vi "grab_video_in_parallel.vi"() -> ()   [LabVIEW 2015]
uses:
  video_global.vi
  <vilib>/LVH/AR Drone Toolkit/AR Drone.lvlib
panel:
  in  "stop 2":bool
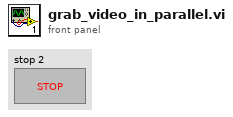
[diagram p1: front panel]
types:
  T1 = typedef "AR Drone.lvlib/AR Drone Resource.ctl" = cluster{"UDP Control Connection":refnum<k16>, "UDP NavData Connection":refnum<k16>, "UDP Video Connection (Drone 1.0)":refnum<k16>, "TCP Video Connection (Drone 2.0)":refnum<k5>, "TCP Control Port Connection":refnum<k5>, "Drone IP address":string, "Drone Command Port":u16, "Drone NavData Port":u16, "Drone Vid Stream Port":u16, "Drone TCP Control Port":u16, "Home IP address":string, "Home Command Port":u16, "Home NavData Port":u16, "Home Vid Stream Port":u16, "Drone Version":i32, "Drone Index":i32, "Command Sequence":i32}
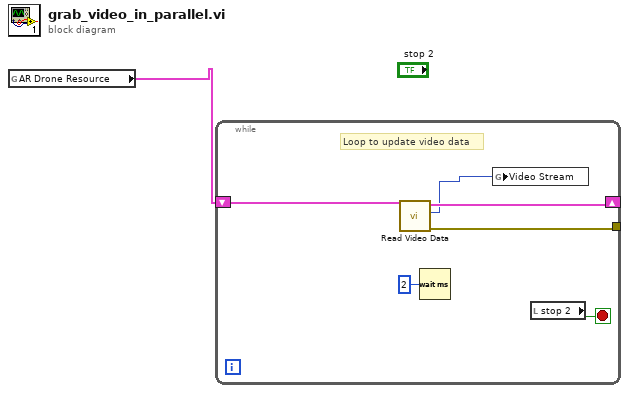
[diagram p0: block diagram]
diagram:
  n1 = global read "video_global.vi" "AR Drone Resource"() -> (w1:T1)
  n2 = while {
    shift-right: [w6] -> _
    shift-left: w1 -> [w7]
    tunnel: [w5] -> _
    stop <- w4 stop-if-true
    # "Loop to update video data"
    n3 = call <vilib>:"Read Video Data.vi"("AR Drone Resource"=w7) -> ("error out"=w5:errorcluster, "Video Stream"=w2:picture, "AR Drone Resource Out"=w6:T1)  [unwired: 8 in]
    n4 = Wait (ms)(milliseconds to wait=u32 2) -> ()  [unwired: 1 out]
    n5 = global write "video_global.vi" "Video Stream"(w2) -> ()
    n6 = local read "stop 2"() -> (w4:bool)
  }
